vi "solar_excel File Write (All).vi"(6 "Visible? (F)":bool, 8 "error in (no error)":errorcluster, 9 "Worksheets Cells":cluster{"Cells":string[][]}[](array[cluster]), 10 "Worksheets":string[](array[string]), 11 "Excel Workbook (*.xlsx)":path) -> (0 "error out":errorcluster, 3 "dup Excel Workbook":path)   [LabVIEW 2018]
doc: "This writes all Worksheets to an Excel Workbook (*.xlsx)."
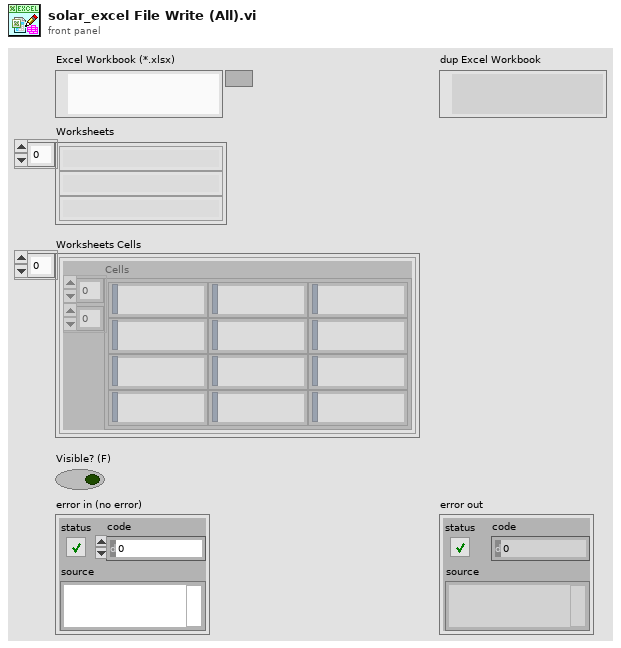
[diagram p1: front panel]
types:
  T1 = typedef "solar_excel_ctl App.ctl" = cluster{"ExcelApp":refnum<k7>, "Workbooks":refnum<k7>, "TSV":refnum<queue>}
  T2 = typedef "solar_excel_ctl Workbook.ctl" = cluster{"ExcelApp":refnum<k7>, "Workbooks":refnum<k7>, "TSV":refnum<queue>, "OpenWkb":refnum<k7>}
  T3 = typedef "solar_excel_ctl Worksheet.ctl" = cluster{"ExcelApp":refnum<k7>, "Workbooks":refnum<k7>, "TSV":refnum<queue>, "OpenWkb":refnum<k7>, "Worksheets":refnum<k7>, "OpenWksh":refnum<k7>}
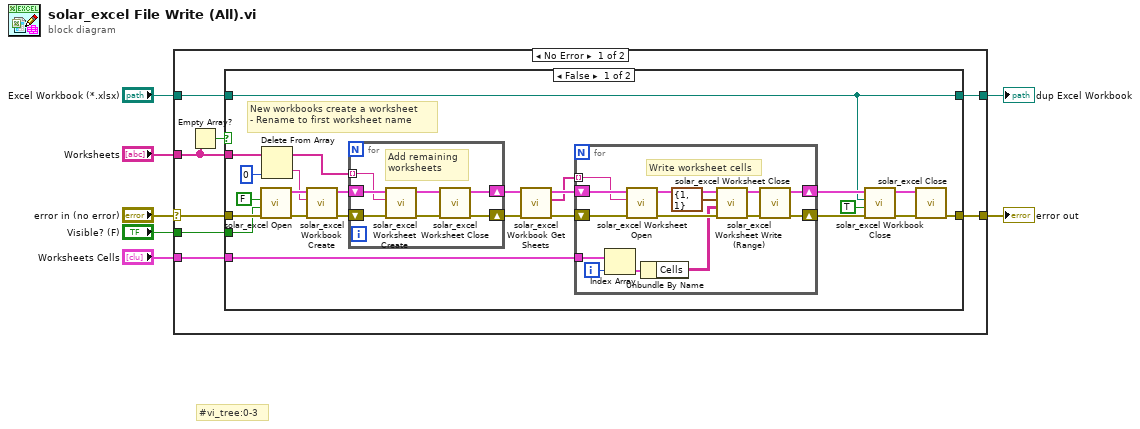
[diagram p0: block diagram]
diagram:
  # "#vi_tree:0-3"
  n1 = case shown="No Error" "error in (no error)" {
    selector: "error in (no error)" -> [w14 w64]
    tunnel: [w15 w64] -> w7
    tunnel: "Visible? (F)" -> [w13 _]
    tunnel: "Excel Workbook (*.xlsx)" -> [w12 w63]
    tunnel: [w8 w63] -> w3
    tunnel: "Worksheets Cells" -> [w11 _]
    tunnel: "Worksheets" -> [w10 _]
    frame No Error {
      n2 = Empty Array?(array=w10) -> (empty?=w9:bool)
      n3 = case shown="False" w9 {
        tunnel: [w39 w61] -> w15
        tunnel: w14 -> [w38 w61]
        tunnel: w13 -> [w37 _]
        tunnel: w10 -> [w29 _]
        tunnel: w12 -> [w16 w62]
        tunnel: w11 -> [w19 _]
        tunnel: [w16 w62] -> w8
        frame False {
          # "New workbooks create a worksheet\n- Rename to first worksheet name"
          n4 = call "solar_excel Open.vi"("error in (no error)"=w38, "Visible? (F)"=w37, "Open New Instance? (F)"=FALSE) -> ("error out"=w35:errorcluster, "Excel App"=w34:T1)  [unwired: 7 in]
          n5 = Delete From Array(array=w29, index=0) -> (deleted portion=w28:string, array with subset deleted=w20:string[])  [unwired: 1 in]
          n6 = call "solar_excel Workbook Create.vi"("error in (no error)"=w35, "Worksheet"=w28, "Excel App"=w34) -> ("error out"=w21:errorcluster, "Excel Workbook"=w23:T2)  [unwired: 7 in]
          n7 = for {
            shift-right: [w55] -> w24
            shift-left: w23 -> [w59]
            shift-right: [w56] -> w22
            shift-left: w21 -> [w60]
            tunnel: w20 -> [w54] mode=indexing
            # "Add remaining\nworksheets"
            n8 = call "solar_excel Worksheet Create.vi"("error in (no error)"=w60, "New Worksheet Name"=w54, "Excel Workbook"=w59) -> ("error out"=w57:errorcluster, "Excel Worksheet"=w58:T3)  [unwired: 7 in]
            n9 = call "solar_excel Worksheet Close.vi"("error in (no error)"=w57, "Excel Worksheet"=w58) -> ("error out"=w56:errorcluster, "Excel Workbook"=w55:T2)  [unwired: 8 in]
          }
          n10 = call "solar_excel Workbook Get Sheets.vi"("error in (no error)"=w22, "Excel Workbook in"=w24) -> ("error out"=w31:errorcluster, "Worksheet Names"=w18:string[], "Excel Workbook out"=w30:T2)  [unwired: 6 in, 1 out]
          n11 = for {
            shift-right: [w50] -> w26
            shift-left: w31 -> [w53]
            shift-right: [w51] -> w27
            shift-left: w30 -> [w52]
            tunnel: w19 -> [w44]
            tunnel: w18 -> [w42] mode=indexing
            i -> [w40]
            # "Write worksheet cells"
            n12 = Index Array(array=w44, index=w40) -> (element=w41:cluster{"Cells":string[][]})
            n13 = call "solar_excel Worksheet Open.vi"("error in (no error)"=w53, "Sheet Name (STR) or Number (I32)"=w42, "Excel Workbook"=w52) -> ("error out"=w46:errorcluster, "Excel Worksheet"=w49:T3)  [unwired: 5 in, 2 out]
            n14 = Unbundle By Name(w41) -> ("Cells"=w43:string[][])
            n15 = call "solar_excel Worksheet Write (Range).vi"("error in (no error)"=w46, "Cells"=w43, "Start (1,1 = 'A1')"=cluster{"Row":u32, "Column":u32} {"Row"=1, "Column"=1}, "Excel Worksheet in"=w49) -> ("error out"=w47:errorcluster, "Excel Worksheet out"=w48:T3)  [unwired: 6 in]
            n16 = call "solar_excel Worksheet Close.vi"("error in (no error)"=w47, "Excel Worksheet"=w48) -> ("error out"=w50:errorcluster, "Excel Workbook"=w51:T2)  [unwired: 8 in]
          }
          n17 = call "solar_excel Workbook Close.vi"("error in (no error)"=w26, "Save? (F)"=TRUE, "Excel Workbook (*.xlsx)"=w16, "Excel Workbook"=w27) -> ("error out"=w33:errorcluster, "Excel App"=w32:T1)  [unwired: 6 in]
          n18 = call "solar_excel Close.vi"("error in (no error)"=w33, "Excel App"=w32) -> ("error out"=w39:errorcluster)  [unwired: 9 in]
        }
        frame True {
          # "Empty Worksheets\n- Do nothing"
        }
      }
    }
    frame Error {
    }
  }
  "error out" <- w7
  "dup Excel Workbook" <- w3
